vi "resolve VI reference.vi"(8 "error in":errorcluster, 11 "VI reference":refnum<vi>) -> (0 "error out":errorcluster, 3 "UI Ref":refnum<vi>)   [LabVIEW 2013, in "UI Reference runtime.lvclass"]
doc: "Opens reference to top-level VI if the provided reference is invalid."
uses:
  UI Reference runtime.lvclass
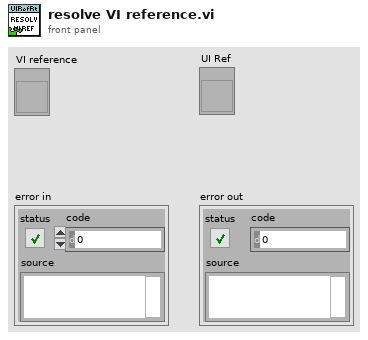
[diagram p1: front panel]
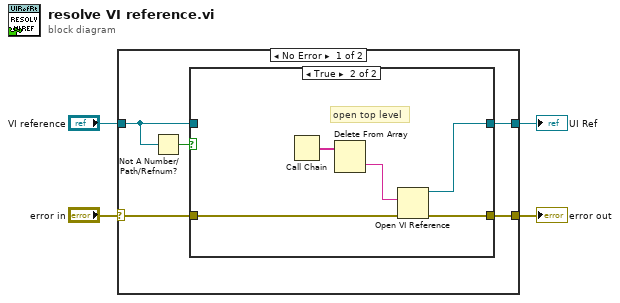
[diagram p0: block diagram]
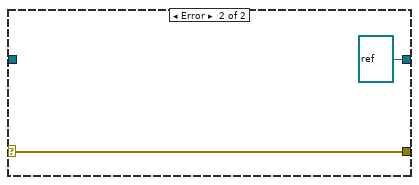
[diagram p3: hidden frame]
diagram:
  n1 = case shown="No Error" "error in" {
    selector: "error in" -> [w5 w18]
    tunnel: "VI reference" -> [w8 _]
    tunnel: [w7 refnum<vi> refnum ("VI reference")] -> w3
    tunnel: [w6 w18] -> w2
    frame No Error {
      n2 = Not A Number/Path/Refnum?(number/path/refnum=w8) -> (NaN/Path/Refnum?=w9:bool)
      n3 = case shown="True" w9 {
        tunnel: w8 -> [w11 _]
        tunnel: [w11 w16] -> w7
        tunnel: w5 -> [w10 w14]
        tunnel: [w10 w15] -> w6
        frame False {
        }
        frame True {
          # "open top level"
          n4 = Call Chain() -> (call chain=w13:string[])
          n5 = Delete From Array(array=w13) -> (deleted portion=w12:string)  [unwired: 2 in, 1 out]
          n6 = Open VI Reference(vi path=w12, error in (no error)=w14) -> (vi reference=w16:refnum<vi>, error out=w15:errorcluster)  [unwired: 4 in]
        }
      }
    }
    frame Error {
    }
  }
  "UI Ref" <- w3
  "error out" <- w2
